vi "Packet Decode.vi"(8 "error in (no error)":errorcluster, 10 "Data":u8[](array[numeric]), 11 "Direction in":refnum<class "Direction.lvclass">) -> (0 "error out":errorcluster, 3 "Direction out":refnum<class "Direction.lvclass">)   [LabVIEW 2019, in "Direction.lvclass"]
uses:
  Direction.lvclass
  Direction STYP.ctl
  PlayerUpdate/PlayerUpdate.lvclass
  TCP Packet/Packet.lvclass
  C:/projects/labview_multiplayer_snake/Main Codeline/Software/Code/Shared/PlayerUpdate/PlayerUpdate.lvclass
  C:/projects/labview_multiplayer_snake/Main Codeline/Software/Code/Shared/TCP/JSONPayload/JSONPayload.lvclass
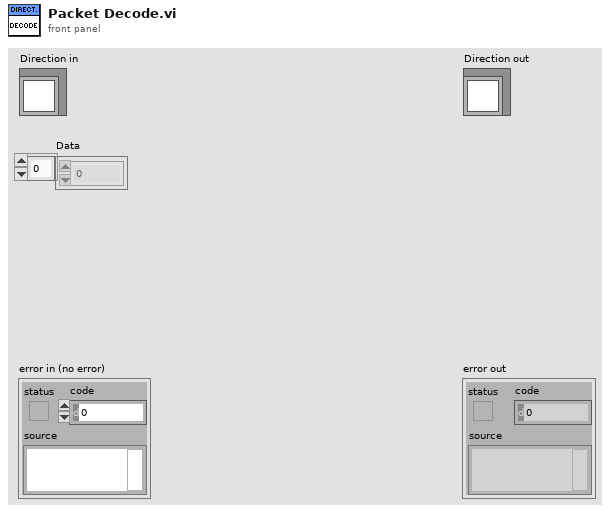
[diagram p1: front panel]
types:
  T1 = typedef "Direction STYP.ctl" = enum16{"Up", "Down", "Left", "Right"}
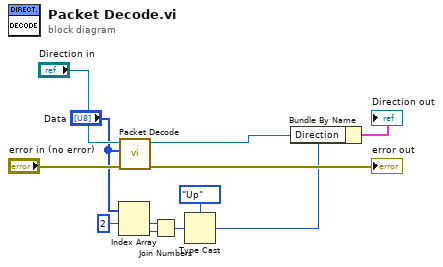
[diagram p0: block diagram]
diagram:
  n1 = Index Array(array="Data", index #1=2 ("index")) -> (element #1=w5:u8, element #2=w4:u8)  [unwired: 1 in]
  n2 = call-parent "Packet Decode.vi"("error in (no error)"="error in (no error)", "Data"="Data", "Packet in"="Direction in") -> ("error out"=→"error out":errorcluster, "Packet out"=w11:refnum<class "Packet.lvclass">)  [unwired: 7 in]
  n3 = Join Numbers(hi=w5, lo=w4) -> ((hi.lo)=w3:u16)
  n4 = Type Cast(type=Direction_STYP."Up" ("Direction"), x=w3) -> (*(type *) &x=w1:T1)
  n5 = Bundle By Name(cluster=w11, "Direction"=w1) -> (→"Direction out":cluster{})
